vi "add Segment.vi"(8 "error in (no error)":errorcluster caption="Fehler (Eingang, kein Fehler)", 10 "Segment.lvclass":refnum<class "Segment.lvclass">, 11 "Test Eingang":refnum<class "Test.lvclass"> caption="Test in") -> (0 "error out":errorcluster caption="Fehler (Ausgang)", 3 "Test Ausgang":refnum<class "Test.lvclass"> caption="Test out")   [LabVIEW 2013, in "DatenKlassen.lvlib" / "Test.lvclass"]
uses:
  Test.lvclass
  Segment/Segment.lvclass
  Test.lvclass/Test.ctl
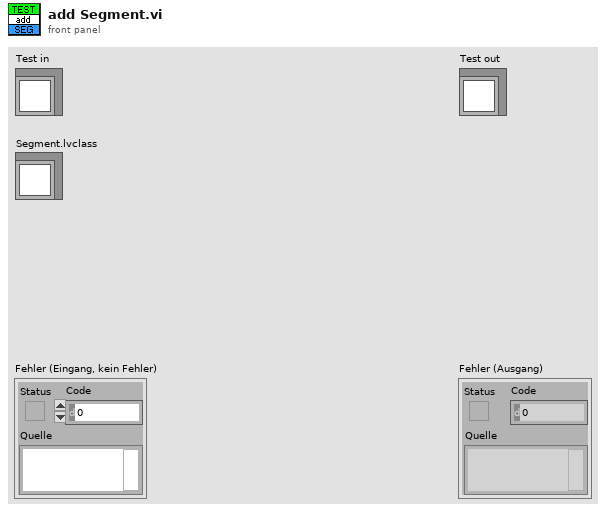
[diagram p1: front panel]
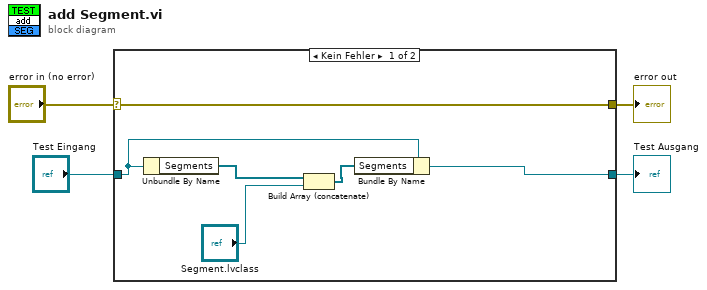
[diagram p0: block diagram]
diagram:
  n1 = case shown="Kein Fehler" "error in (no error)" {
    selector: "error in (no error)" -> [w10 w12]
    tunnel: [w10 w12] -> w3
    tunnel: [w8 w11] -> w1
    tunnel: "Test Eingang" -> [w9 w11]
    frame No Error {
      n2 = Unbundle By Name(w9) -> ("Segments"=w7:refnum<class "Segment.lvclass">[])
      n3 = Build Array (concatenate)(w7, "Segment.lvclass") -> (w5:refnum<class "Segment.lvclass">[])
      n4 = Bundle By Name(cluster=w9, "Segments"=w5) -> (w8:refnum<class "Test.lvclass">)
    }
    frame Error {
    }
  }
  "error out" <- w3
  "Test Ausgang" <- w1
